vi "COMI Read Mem Port DW.vi"(9 "nOffset":u32, 10 "dwPortBase":u32, 11 "hDevice":u32) -> (2 "function return":u32, 3 "hDevice out":u32)   [LabVIEW 2017, in "Comidll.lvlib"]
doc: "unsigned long (COMI_ReadMemPortDW) (HANDLE hDevice, unsigned long dwPortBase, unsigned long nOffset);"
uses:
  <userlib>/Comidll/Comidll.lvlib
  <userlib>/Comidll/Comidll.dll
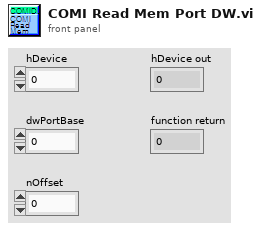
[diagram p1: front panel]
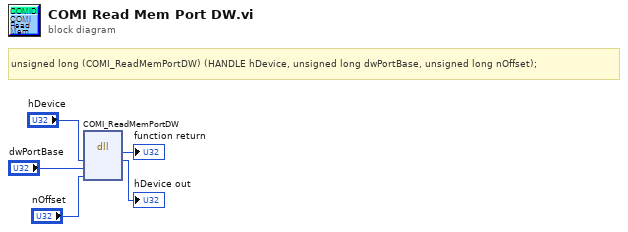
[diagram p0: block diagram]
diagram:
  # "unsigned long\t(COMI_ReadMemPortDW) (HANDLE hDevice, unsigned long dwPortBase, unsigned long nOffset);"
  n1 = dll-call lib="C:/Program Files/National Instruments/LabVIEW 2017/user.lib/Comidll/Comidll.*" fn="COMI_ReadMemPortDW"("hDevice"="hDevice", "dwPortBase"="dwPortBase", "nOffset"="nOffset") -> (→"function return":u32, "hDevice"=→"hDevice out":u32)  [unwired: 5 in, 2 out]
